vi "oef14.vi"() -> ()   [LabVIEW 2021]
panel:
  out "Waveform Graph":dbl[][](graph)
  out "Waveform Chart":cluster{"y":dbl, "y":dbl}(graph)
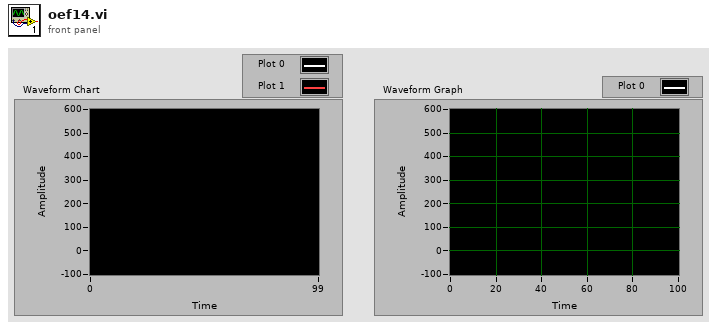
[diagram p1: front panel]
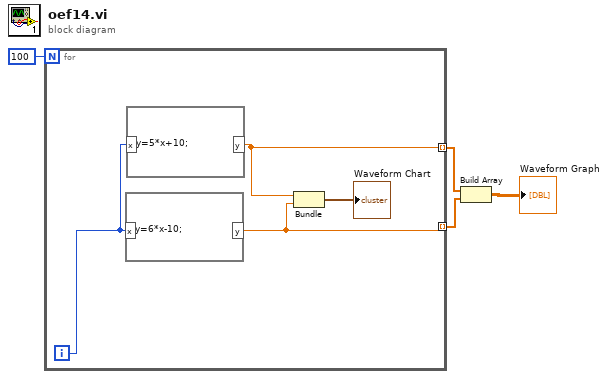
[diagram p0: block diagram]
diagram:
  n1 = for {
    N: 100 -> [_]
    tunnel: [w6] -> w2 mode=indexing
    tunnel: [w5] -> w1 mode=indexing
    i -> [w8]
    n2 = formula code="y=6*x-10;"("x"=w8) -> ("y"=w5:dbl)
    n3 = formula code="y=5*x+10;"("x"=w8) -> ("y"=w6:dbl)
    n4 = Bundle("y"=w6, "y"=w5) -> (→"Waveform Chart":cluster{"y":dbl, "y":dbl})  [unwired: 1 in]
  }
  n5 = Build Array(w2, w1) -> (→"Waveform Graph":dbl[][])
